vi "pre_scan.vi"(6 "scan_values":dbl[](array[numeric]), 7 "override":bool, 8 "error in (no error)":errorcluster, 11 "VISA IN":refnum<visa-resource-name>) -> (0 "error out":errorcluster)   [LabVIEW 2017, in "radiant.lvlib"]
uses:
  radiant.lvlib
panel:
  out "VISA resource out":refnum<visa-resource-name>="COM9"
  in  "VISA (default)":refnum<visa-resource-name>="COM9"
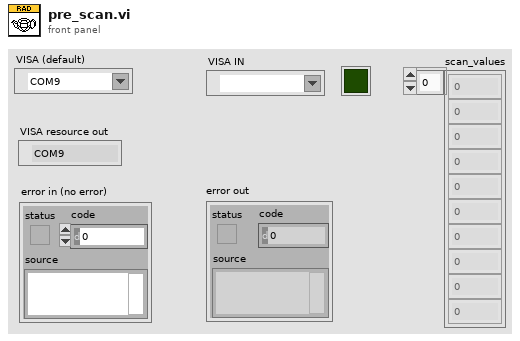
[diagram p1: front panel]
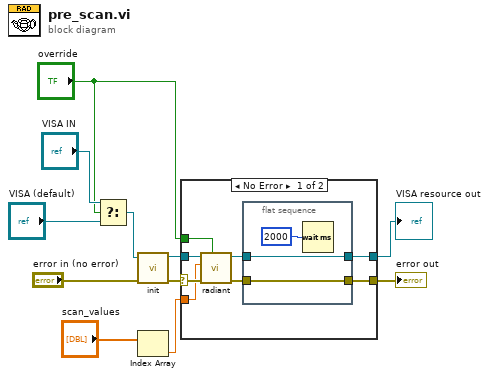
[diagram p0: block diagram]
diagram:
  n1 = Select(t="VISA IN", s="override", f="VISA (default)") -> (s? t:f=w9:refnum<visa-resource-name>)
  n2 = call "init.vi"("error in (no error)"="error in (no error)", "VISA resource name"=w9) -> ("error out"=w7:errorcluster, "VISA resource name out"=w3:refnum<visa-resource-name>)  [unwired: 7 in, 1 out]
  n3 = Index Array(array="scan_values") -> (element=w4:dbl)  [unwired: 1 in]
  n4 = case shown="No Error" w7 {
    selector: w7 -> [w19 w24]
    tunnel: [w15 w24] -> w5
    tunnel: w4 -> [w18 _]
    tunnel: w3 -> [w17 w23]
    tunnel: "override" -> [w16 _]
    tunnel: [w13 w23] -> w1
    frame No Error {
      n5 = call "radiant.vi"("override"=w16, "error in (no error)"=w19, "WL (nm)"=w18, "VISA IN"=w17) -> ("error out"=w14:errorcluster, "VISA resource out"=w12:refnum<visa-resource-name>)  [unwired: 5 in, 1 out]
      n6 = flat-sequence {
        tunnel: [w22] -> w15
        tunnel: w14 -> [w22]
        tunnel: [w20] -> w13
        tunnel: w12 -> [w20]
        frame #0 {
          n7 = Wait (ms)(milliseconds to wait=u32 2000) -> ()  [unwired: 1 out]
        }
      }
    }
    frame Error {
    }
  }
  "error out" <- w5
  "VISA resource out" <- w1
